vi "sub UI get title.vi"(8 "error in (no error)":errorcluster, 11 "IDE simple in":refnum<class "LF2R IDE.lvclass">) -> (0 "error out":errorcluster, 2 "frame title":T1, 3 "IDE simple out":refnum<class "LF2R IDE.lvclass">)   [LabVIEW 2018, in "LF2R IDE.lvlib" / "LF2R IDE.lvclass"]
uses:
  LF2R IDE.lvclass
  Frame Analizer/frame title.ctl
  LF2R IDE.lvclass/LF2R IDE.ctl
  Frame Analizer/Frame Analizer.lvclass
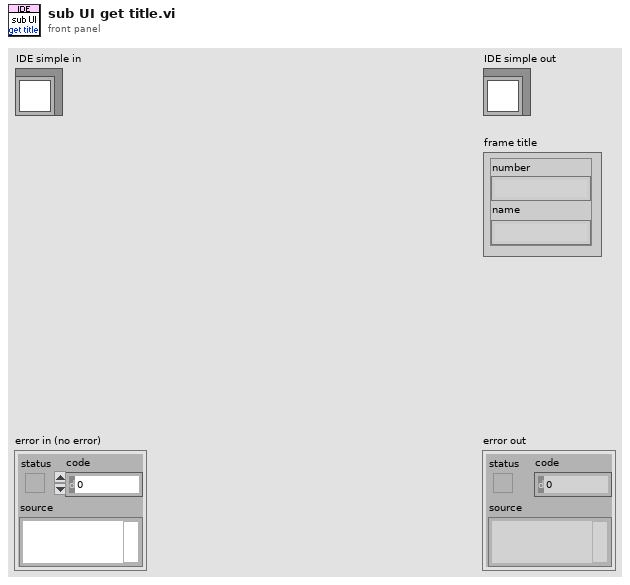
[diagram p1: front panel]
types:
  T1 = typedef "Frame Analizer.lvclass/frame title.ctl" = cluster{"number":string, "name":string}
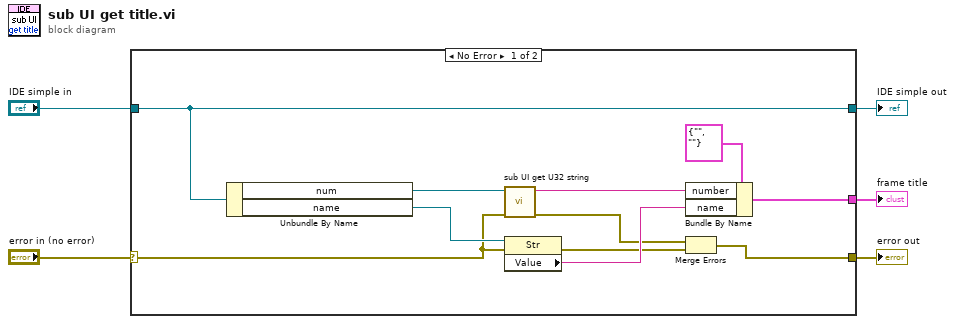
[diagram p0: block diagram]
diagram:
  n1 = case shown="No Error" "error in (no error)" {
    selector: "error in (no error)" -> [w6 w18]
    tunnel: [w15 w18] -> w4
    tunnel: [w16 w17] -> w2
    tunnel: "IDE simple in" -> [w16 w17]
    tunnel: [w14 _] -> w1
    frame No Error {
      n2 = Unbundle By Name(w16) -> ("num"=w12:refnum<vi>, "name"=w10:refnum<vi>)
      n3 = call "sub UI get U32 string.vi"("error in (no error)"=w6, "U32 Ref"=w12) -> ("error out"=w8:errorcluster, "Value string"=w11:string)  [unwired: 8 in]
      n4 = property class="Str"(reference=w10, error in=w6) -> (error out=w7:errorcluster, "Value"=w9:string)  [unwired: 1 out]
      n5 = Bundle By Name(cluster=T1 {"number"="", "name"=""} ("frame title 2"), "number"=w11, "name"=w9) -> (w14:T1)
      n6 = Merge Errors(w8, w7) -> (w15:errorcluster)
    }
    frame Error {
    }
  }
  "error out" <- w4
  "IDE simple out" <- w2
  "frame title" <- w1
